vi "Select Model v0.1.vi"() -> (1 "Cancel out":bool, 2 "Refresh Indicators?":bool, 3 "Model out":string)   [LabVIEW 2021]
uses:
  Controls/Logging FGV.ctl
panel:
  in  "New Shift":bool
  out "Reject Count":u32
  out "Total Count":u32
  out "OEE 2":T1 caption="Latest Measurements" {"AVL" format="%#.1f"; "PRF" format="%#.1f"; "QUA" format="%#.1f"; "OEE" format="%#.1f"}
  out "Timestamp":string caption="Start Time"
  out "PDT (Hr)":dbl caption="Planned Down Time (Hours)"
  out "SPT (Hr)":dbl caption="Scheduled Production Time (Hours)"
  in  "Model":string(combo)="Model A:188.9"
  in  "Cancel Button":bool
  in  "Continue":bool
  # "Please select the Model that you wish to run"
  # "Previous Shift Information"
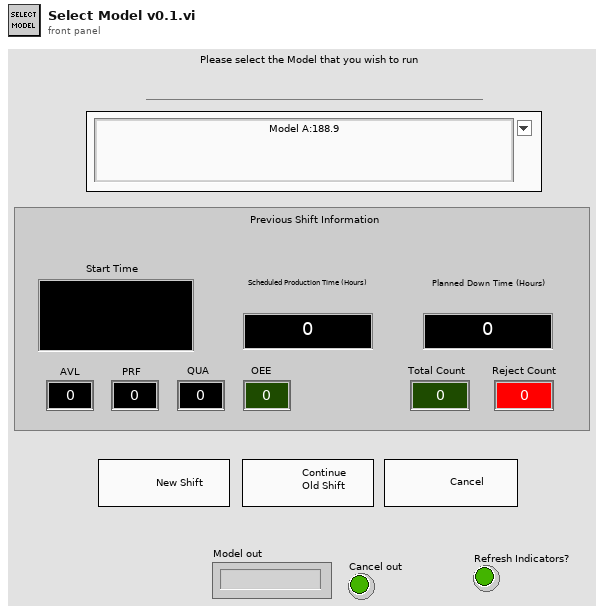
[diagram p1: front panel]
types:
  T1 = cluster{"AVL":dbl, "PRF":dbl, "QUA":dbl, "OEE":dbl}
  T2 = typedef "Logging FGV.ctl" = enum16{"Start Shift", "Reload Values", "Log Index", "Read Shift", "Close Shift", "Save Values"}
  T3 = cluster{"Time-Stamp":timestamp, "Scheduled Time":dbl, "Planned Downtime":dbl}
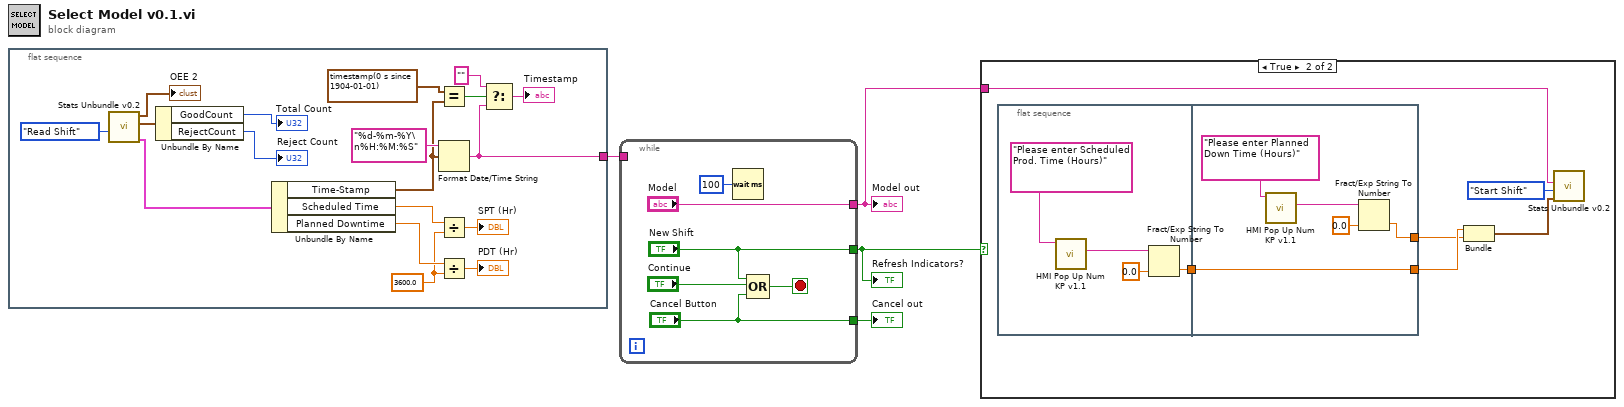
[diagram p0: block diagram]
diagram:
  n1 = flat-sequence {
    tunnel: [w7] -> w3
    frame #0 {
      w18 = 3600.0 ("y")
      n2 = call "Stats Unbundle v0.2.vi"("State"=Logging_FGV."Read Shift") -> ("NAT Cluster out"=w21:T3, "Counters"=w14:cluster{"GoodCount":u32, "RejectCount":u32}, "OEE Cluster"=→"OEE 2":T1)  [unwired: 4 in, 4 out]
      n3 = Unbundle By Name(w14) -> ("GoodCount"=→"Total Count":u32, "RejectCount"=→"Reject Count":u32)
      n4 = Unbundle By Name(w21) -> ("Time-Stamp"=w10:timestamp, "Scheduled Time"=w20:dbl, "Planned Downtime"=w19:dbl)
      n5 = Equal?(x=timestamp(0 s since 1904-01-01) ("Time-Stamp"), y=w10) -> (x = y?=w8:bool)
      n6 = Format Date/Time String(time format string (%c)="%d-%m-%Y\n%H:%M:%S", seconds (now)=w10) -> (date/time string=w7:string)  [unwired: 1 in]
      n7 = Divide(x=w20, y=w18) -> (x/y=→"SPT (Hr)":dbl)
      n8 = Divide(x=w19, y=w18) -> (x/y=→"PDT (Hr)":dbl)
      n9 = Select(t="", s=w8, f=w7) -> (s? t:f=→"Timestamp":string)
    }
  }
  n10 = while {
    tunnel: ["Model"] -> w1
    tunnel: ["Cancel Button"] -> w4
    tunnel: ["New Shift"] -> w2
    tunnel: w3 -> [_]
    stop <- w27 stop-if-true
    n11 = Wait (ms)(milliseconds to wait=u32 100) -> ()  [unwired: 1 out]
    n12 = Compound Arithmetic op=OR("New Shift", "Continue", "Cancel Button") -> (w27:bool)
  }
  "Model out" <- w1
  "Cancel out" <- w4
  "Refresh Indicators?" <- w2
  n13 = case shown="True" w2 {
    tunnel: w1 -> [_ w29]
    frame False {
    }
    frame True {
      n14 = flat-sequence {
        tunnel: [w35] -> w34
        tunnel: [w40] -> w32
        tunnel: w34 -> [w40]
        tunnel: [w39] -> w30
        frame #0 {
          n15 = call "HMI Pop Up Num KP v1.1.vi"("Message In"="Please enter Scheduled Prod. Time (Hours)") -> ("String Out"=w36:string)  [unwired: 9 in, 1 out]
          n16 = Fract/Exp String To Number(string=w36, default (0 dbl)=0.0 ("default (0 I32)")) -> (number=w35:dbl)  [unwired: 2 in, 1 out]
        }
        frame #1 {
          n17 = call "HMI Pop Up Num KP v1.1.vi"("Message In"="Please enter Planned Down Time (Hours)") -> ("String Out"=w43:string)  [unwired: 9 in, 1 out]
          n18 = Fract/Exp String To Number(string=w43, default (0 dbl)=0.0 ("default (0 I32)")) -> (number=w39:dbl)  [unwired: 2 in, 1 out]
        }
      }
      n19 = Bundle(w32, w30) -> (w31:cluster{dbl, dbl})  [unwired: 1 in]
      n20 = call "Stats Unbundle v0.2.vi"("NAT Cluster in"=w31, "State"=Logging_FGV."Start Shift", "Model"=w29) -> ()  [unwired: 2 in, 7 out]
    }
  }
